vi "CRYGet Curve & ProtectName.vi"(9 "Type In":enum16{"Curves", "Values", "Results", "WFM"}(ring), 10 "FlattenData":string, 11 "Category":string) -> (3 "NameOut":string[](array[string]))   [LabVIEW 2013]
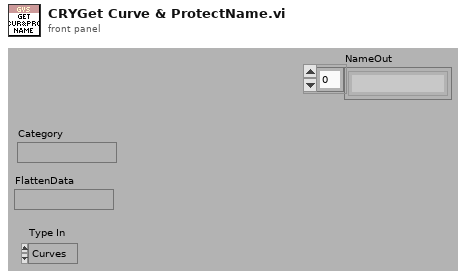
[diagram p1: front panel]
types:
  T1 = cluster{"StepName":string, "setup flattened":string}[]
  T2 = typedef "CRYStimulus Cluster.ctl" = cluster{"StimulusType":string, "UseMLValArray":u16[], "ML_axisArray":u16[], "MLValLevelNameArray":string[], "Level(U)Array":dbl[], "Start(Stop)FreqArray":dbl[], "Start(Stop)AmpArray":dbl[], "StepResolutionArray":u16[], "Unit_Array":u16[], "DegValArray":dbl[], "DegUnitArray":string[], "Steps1":i32, "Cycle/step1(#)":u32, "Time/step1(s)":dbl, "Transition1":dbl, "SweepRate2":dbl, "Freq3(Hz)":dbl, "Steps3(#)":dbl, "Cycles3(#)":u32, "StepSize3":dbl, "wave time":string, "RMS_Value4":dbl, "Peak_Value4":dbl, "WavePath4":string, "RMS_unit4":string, "Peak_unit4":string, "wave Info":string, "dc_ctrl5_1":u16, "dc_ctrl5_2":u16, "dc_polar5":u16, "Max.Current":u16, "Steps5(#)":u32, "Time/Step5":dbl, "Level5":dbl, "StepsSize5Val":dbl, "StepSize5Unit":string, "SweepType":u16, "Fixed/Ratio6":u16, "Transition6":dbl, "Steps6(#)":dbl, "Cycle/Steps6(#)":u32, "Time/Steps6(s)":dbl, "Freq6(Hz)":dbl, "Difference6(Hz)":dbl, "Ratio6":string, "NoiseType7":u16, "Duration7(s)":dbl, "MinFreq7(Hz)":dbl, "MaxFreq7(Hz)":dbl, "MinFreq8(Hz)":dbl, "MaxFreq8(Hz)":dbl, "FreqRounding8":bool, "Duration8(s)":dbl, "Tones8":dbl, "RoundingVal8":dbl, "ApplyEQ":bool, "Duration(s)":dbl, "CustomStimulusName ":string, "Flatten Element Array":string[], "sine waves":cluster{"freq":dbl, "ampl":dbl, "cycles":dbl}[], "Channel Out":i32, "RatioVal6":dbl, "TabCtrl6":enum32{"Master Tone", "Slave Tone"}, "Signal Type Name":string, "Help":string, "Channel Sel":u16}
  T3 = typedef "CRYWaveform Cluster Array.ctl" = T4[]
  T4 = typedef "CRYWaveform Cluster.ctl" = cluster{"Waveform":cluster{"X0":dbl, "dX":dbl, "Y":sgl[]}, "X data":u16, "Y data":u16, "Y axis":u16, "X unit":string, "Y unit":string, "Y dB ref":dbl, "display Y":bool, "display X":bool, "Overload?":bool, "Test Info":string, "Step No.":i32, "Name":string, "protected":bool, "Sqc history":string[], "Signal Channel ID":i32, "Plot Settings":cluster{"Color":u32, "Interpolation":u8, "Point Style":u8, "Line Style":u8, "Point Color":u32, "Line Width":u8, "Bar Plot Style":u8, "Fill To":i16}, "AutoProtect":bool}
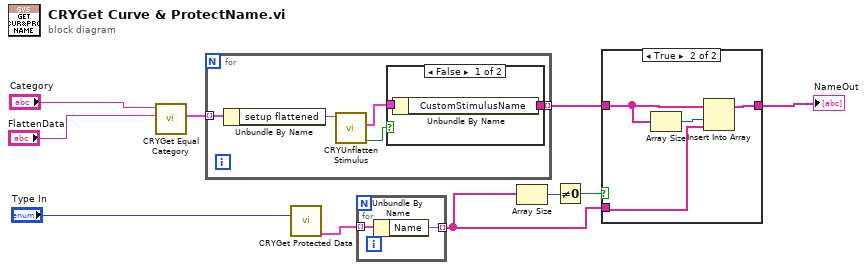
[diagram p0: block diagram]
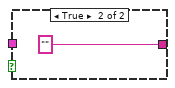
[diagram p3: hidden frame]
diagram:
  n1 = call "CRYGet Equal Category.vi"("Current StepName"="FlattenData", "Find CategoryName"="Category") -> ("setup flattened Array out"=w5:T1)  [unwired: 9 out]
  n2 = for {
    tunnel: w5 -> [w15] mode=indexing
    tunnel: [w11] -> w6 mode=indexing
    n3 = Unbundle By Name(w15) -> ("setup flattened"=w14:string)
    n4 = call "CRYUnflatten Stimulus.vi"("Flatten Stimulus"=w14) -> ("Error?"=w13:bool, "Stimulus"=w12:T2)  [unwired: 9 out]
    n5 = case shown="False" w13 {
      tunnel: w12 -> [w17 _]
      tunnel: [w16 "" ("CustomStimulusName")] -> w11
      frame False {
        n6 = Unbundle By Name(w17) -> ("CustomStimulusName"=w16:string)
      }
      frame True {
      }
    }
  }
  n7 = call "CRYGet Protected Data.vi"("Type In"="Type In") -> ("Waveform Array"=w9:T3)  [unwired: 10 out]
  n8 = for {
    tunnel: w9 -> [w20] mode=indexing
    tunnel: [w19] -> w10 mode=indexing
    n9 = Unbundle By Name(w20) -> ("Name"=w19:string)
  }
  n10 = Array Size(array=w10) -> (size(s)=w7:i32)
  n11 = Not Equal To 0?(x=w7) -> (x != 0?=w8:bool)
  n12 = case shown="True" w8 {
    tunnel: w6 -> [w21 w22]
    tunnel: [w21 w24] -> w1
    tunnel: w10 -> [_ w25]
    frame False {
    }
    frame True {
      n13 = Array Size(array=w22) -> (size(s)=w23:i32)
      n14 = Insert Into Array(array=w22, index=w23, new element=w25) -> (w24:string[])
    }
  }
  "NameOut" <- w1
